vi "WinCI Find All Providers.vi"(8 "error in (no error)":errorcluster) -> (0 "error out":errorcluster, 1 "additional data":string[](array[string]), 2 "provider locations":string[](array[string]), 3 "provider names":string[](array[string]))   [LabVIEW 2017, in "NI_SCC_WinCI.lvlib"]
uses:
  <vilib>/SourceControl/Providers/WinCI/NI_SCC_WinCI.lvlib
  <vilib>/registry/registry.llb/Registry RtKey.ctl
  <vilib>/registry/registry.llb/Registry SAM.ctl
  <vilib>/registry/registry.llb/Read Registry Value Simple STR.vi
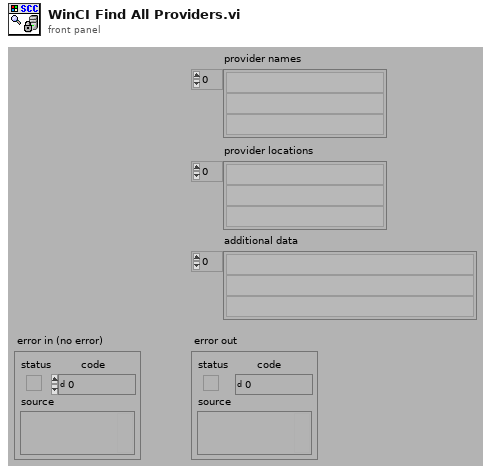
[diagram p1: front panel]
types:
  T1 = typedef "Registry SAM.ctl" = enum32{"KEY_QUERY_VALUE", "KEY_SET_VALUE", "KEY_CREATE_SUB_KEY", "KEY_ENUMERATE_SUB_KEYS", "KEY_NOTIFY", "KEY_CREATE_LINK", "KEY_READ", "KEY_WRITE", "KEY_ALL_ACCESS", "KEY_READ | KEY_WRITE"}
  T2 = typedef "Registry RtKey.ctl" = enum32{"HKEY_CLASSES_ROOT", "HKEY_CURRENT_USER", "HKEY_LOCAL_MACHINE", "HKEY_USERS", "HKEY_PERFORMANCE_DATA", "HKEY_CURRENT_CONFIG", "HKEY_DYN_DATA"}
  T3 = typedef "Registry refnum.ctl" = refnum<k1>
  T4 = cluster{"numValues":i32, "maxValueNameLen":i32, "maxValueDataLen":i32}
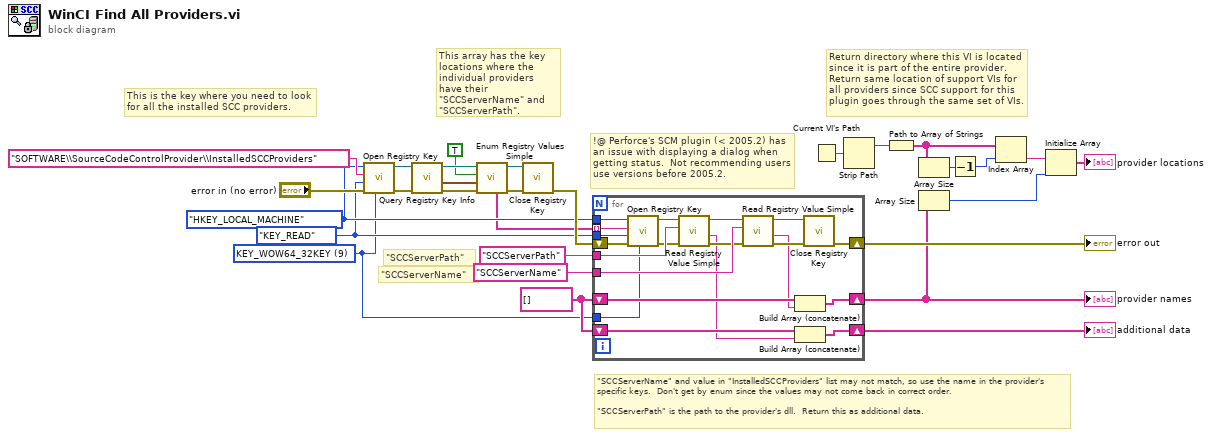
[diagram p0: block diagram]
diagram:
  w1 = u16 9 items=["DEFAULT"=0, "KEY_WOW64_64KEY"=8, "KEY_WOW64_32KEY"=9] ("alternate registry view mask")
  w2 = string[] []
  w10 = Registry_SAM."KEY_READ" ("security access mask (KEY_READ | KEY_WRITE)")
  w11 = Registry_RtKey."HKEY_LOCAL_MACHINE" ("root key (HKEY_LOCAL_MACHINE)")
  # "!@ Perforce's SCM plugin (< 2005.2) has an issue with displaying a dialog when getting status.  Not recommending users use versions before 2005.2."
  # "\"SCCServerName\" and value in \"InstalledSCCProviders\" list may not match, so use the name in the provider's specific keys.  Don't get by enum since the values may not come back in correct order.  \n\n\"SCCServerPath\" is the path to the provider's dll.  Return this as additional data."
  # "\"SCCServerPath\""
  # "\"SCCServerName\""
  # "This array has the key locations where the individual providers have their \"SCCServerName\" and \"SCCServerPath\"."
  # "Return directory where this VI is located since it is part of the entire provider.  Return same location of support VIs for all providers since SCC support for this plugin goes through the same set of VIs."
  # "This is the key where you need to look for all the installed SCC providers."
  n1 = call <vilib>:"Open Registry Key.vi"("registry view"=w1, "error in (no error)"="error in (no error)", "security access mask (KEY_READ | KEY_WRITE)"=w10, "subkey"="SOFTWARE\\SourceCodeControlProvider\\InstalledSCCProviders", "root key (HKEY_LOCAL_MACHINE)"=w11) -> ("error out"=w22:errorcluster, "refnum out"=w21:T3)  [unwired: 5 out]
  n2 = call <vilib>:"Query Registry Key Info.vi"("error in (no error)"=w22, "refnum"=w21) -> ("error out"=w24:errorcluster, "value info"=w25:T4, "refnum out"=w23:T3)  [unwired: 7 out]
  n3 = call <vilib>:"Enum Registry Values Simple.vi"("error in (no error)"=w24, "value info"=w25, "retrieve data? (F)"=TRUE, "refnum"=w23) -> ("error out"=w27:errorcluster, "refnum out"=w26:T3, "String/Binary data"=w8:string[])  [unwired: 5 out]
  n4 = call <vilib>:"Close Registry Key.vi"("error in (no error)"=w27, "refnum"=w26) -> ("error out"=w12:errorcluster)  [unwired: 5 out]
  n5 = for {
    shift-right: [w46] -> w7
    shift-left: w12 -> [w49]
    tunnel: w11 -> [w48]
    tunnel: w8 -> [w41] mode=indexing
    tunnel: w10 -> [w47]
    tunnel: "SCCServerPath" ("string/binary data") -> [w45]
    tunnel: "SCCServerName" ("string/binary data") -> [w44]
    shift-right: [w43] -> w3
    shift-left: w2 -> [w40]
    shift-right: [w42] -> w4
    shift-left: w2 -> [w39]
    tunnel: w1 -> [w30]
    n6 = call <vilib>:"Open Registry Key.vi"("registry view"=w30, "error in (no error)"=w49, "security access mask (KEY_READ | KEY_WRITE)"=w47, "subkey"=w41, "root key (HKEY_LOCAL_MACHINE)"=w48) -> ("error out"=w35:errorcluster, "refnum out"=w38:T3)  [unwired: 5 out]
    n7 = call-poly <vilib>:"Read Registry Value Simple.vi"("error in (no error)"=w35, "value"=w45, "refnum"=w38) -> ("error out"=w36:errorcluster, "String/Binary data"=w31:string, "refnum out"=w37:T3)  [unwired: 1 in, 3 out]
    n8 = call-poly <vilib>:"Read Registry Value Simple.vi"("error in (no error)"=w36, "value"=w44, "refnum"=w37) -> ("error out"=w34:errorcluster, "String/Binary data"=w32:string, "refnum out"=w33:T3)  [unwired: 1 in, 3 out]
    n9 = Build Array (concatenate)(w40, w32) -> (w43:string[])
    n10 = Build Array (concatenate)(w39, w31) -> (w42:string[])
    n11 = call <vilib>:"Close Registry Key.vi"("error in (no error)"=w34, "refnum"=w33) -> ("error out"=w46:errorcluster)  [unwired: 5 out]
  }
  "error out" <- w7
  "provider names" <- w3
  "additional data" <- w4
  n12 = Current VI's Path() -> (path=w18:path)
  n13 = Strip Path(path=w18) -> (stripped path=w17:path)  [unwired: 1 out]
  n14 = Path to Array of Strings(0:w17) -> (2:w15:string[])  [unwired: 1 out]
  n15 = Array Size(array=w15) -> (size(s)=w16:i32)
  n16 = Array Size(array=w3) -> (size(s)=w19:i32)
  n17 = Decrement(x=w16) -> (x-1=w14:i32)
  n18 = Index Array(array=w15, index=w14) -> (element=w13:string)
  n19 = Initialize Array(w13, w19) -> (→"provider locations":string[])
